vi "Semaphore Wait.vi"(8 "error in (no error)":errorcluster, 11 "Semaphore in":T1) -> (0 "error out":errorcluster, 3 "Semaphore out":T1)   [LabVIEW 2013, in "POSIX Threads.lvlib" / "Semaphore.lvclass"]
doc: "Calls sem_wait() on the semaphore object encapsulated by Semaphore.\n\nThis VI decrements the value of the semaphore by 1. However, it can only decrement if the semaphore value is above 0. If the semaphore's value is already greater than zero, this function decrements the semaphore by 1 and returns immediately. If the count is equal to zero, this VI waits indefinitely for the semaphore's value to increment to a value greater than 0, and then attempts to decrement the semaphore and return.\n\nRefer to online POSIX documentation for more information."
uses:
  Semaphore.lvclass
  Controls/reference.ctl
  POSIX Thread Object/POSIX Thread Object.lvclass/POSIX Thread Object.ctl
  POSIX Thread Object/Private VIs/libpthread path.vi
  POSIX Thread Object/Private VIs/get pthread error.vi
  <vilib>/NI/NI Linux RT Errno/VIs/Public/SubVIs/errno enum to number.vi
  <vilib>/NI/NI Linux RT Errno/VIs/Public/Get Errno Value for Calling Thread.vi
  POSIX Thread Object/POSIX Thread Object.lvclass
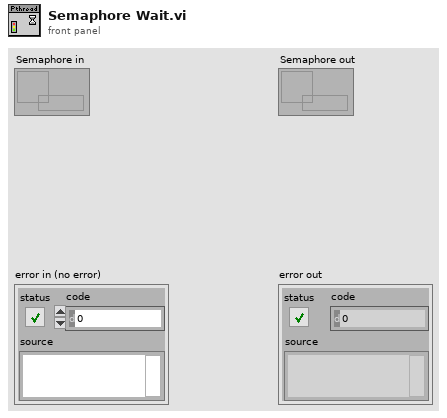
[diagram p1: front panel]
types:
  T1 = typedef "POSIX Threads.lvlib/Semaphore.lvclass/reference.ctl" = refnum<data-value>
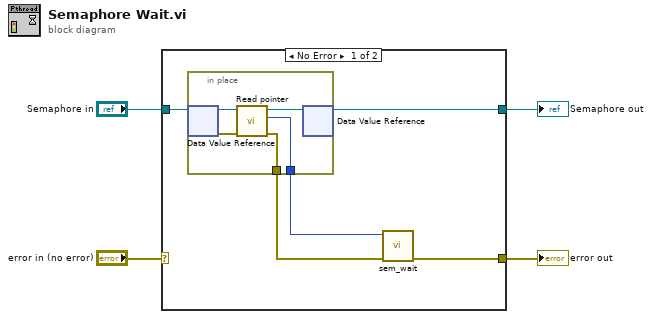
[diagram p0: block diagram]
diagram:
  n1 = case shown="No Error" "error in (no error)" {
    selector: "error in (no error)" -> [_ w15]
    tunnel: "Semaphore in" -> [w9 w16]
    tunnel: [w8 w16] -> w1
    tunnel: [w7 w15] -> w2
    frame No Error {
      n2 = in-place {
        in-place-border: [w11] -> w6
        in-place-border: [w10] -> w5
        n3 = in-place-dvr #1(w9) -> (w14:refnum<class "Semaphore.lvclass">, w13:errorcluster)
        n4 = call "Read pointer.vi"("error in (no error)"=w13, "POSIX Thread Object in"=w14) -> ("error out"=w11:errorcluster, "pointer"=w10:u64, "POSIX Thread Object out"=w12:refnum<class "Semaphore.lvclass">)  [unwired: 7 in]
        n5 = in-place-dvr #1(w12) -> (w8:T1)  [unwired: 1 out]
      }
      n6 = call "sem_wait.vi"("error in (no error)"=w6, "sempahore ptr in"=w5) -> ("error out"=w7:errorcluster)  [unwired: 8 in, 1 out]
    }
    frame Error {
    }
  }
  "error out" <- w2
  "Semaphore out" <- w1
